vi "Typecase.vi"() -> ()   [LabVIEW 2022 SP3]
panel:
  out "*(type *) &x":string
  out "appended array":string[](array[string])
  out "String 2":string
  in  "String":string
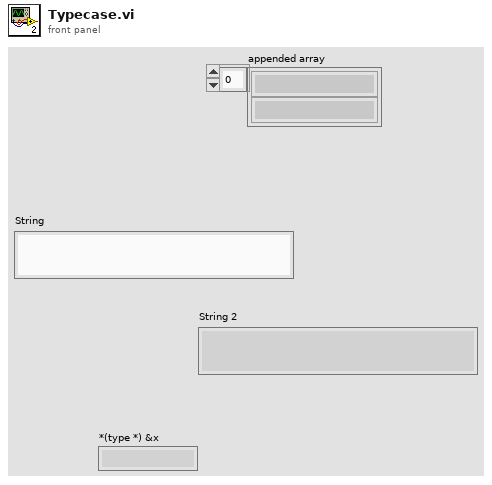
[diagram p1: front panel]
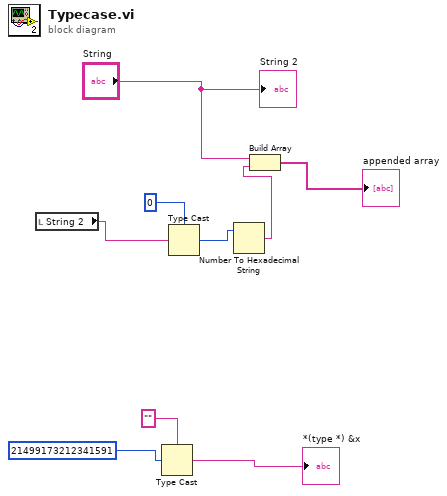
[diagram p0: block diagram]
diagram:
  n1 = local read "String 2"() -> (w7:string)
  n2 = Type Cast(type="", x=i64 21499173212341591) -> (*(type *) &x=→"*(type *) &x":string)
  n3 = Type Cast(type=i64 0, x=w7) -> (*(type *) &x=w5:i64)
  n4 = Number To Hexadecimal String(2:w5) -> (0:w4:string)  [unwired: 1 in]
  n5 = Build Array("String", w4) -> (→"appended array":string[])
  "String 2" <- "String"
